vi "askForSerialNumber.vi"() -> (1 "Stop":bool, 2 "Setup":bool, 3 "Serial Number scanned":string)   [LabVIEW 2013]
panel:
  in  "Serial Number":string
  in  "OK Button":bool
  in  "Stop":bool
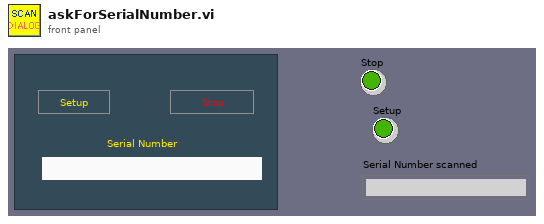
[diagram p1: front panel]
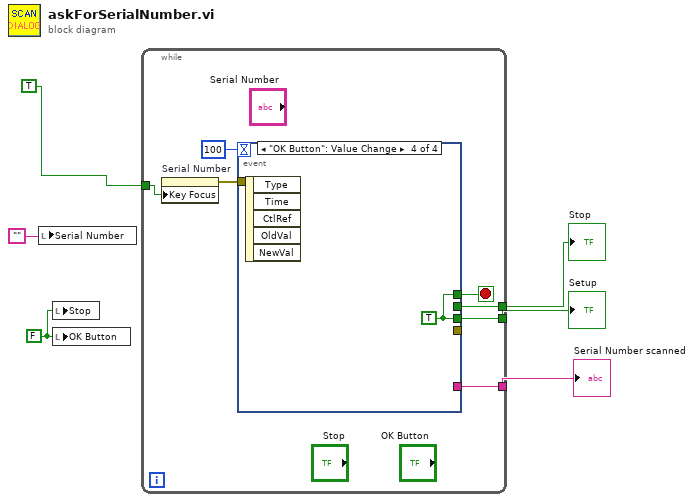
[diagram p0: block diagram]
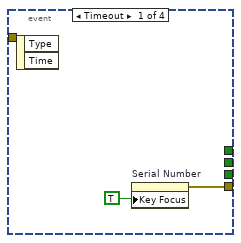
[diagram p2: hidden frame]
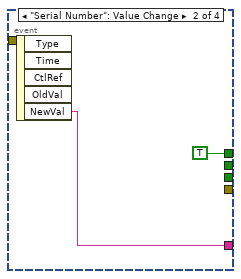
[diagram p3: hidden frame]
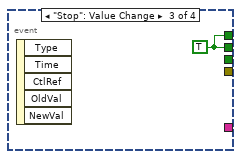
[diagram p4: hidden frame]
diagram:
  w4 = FALSE
  n1 = local write "Serial Number"("") -> ()
  n2 = local write "Stop"(w4) -> ()
  n3 = local write "OK Button"(w4) -> ()
  n4 = while {
    tunnel: [w12] -> w3
    tunnel: [w11] -> w6
    tunnel: [w10] -> w5
    tunnel: TRUE -> [w7]
    stop <- w9 stop-if-true
    n5 = property on="Serial Number" class="Str"("Key Focus"=w7) -> (error out=w8:errorcluster)  [unwired: 2 in, 1 out]
    n6 = event shown="[3] \"OK Button\": Value Change" {
      selector: _ -> [_ _ _ _]
      dyn-events: _ -> [_ _ _ _]
      timeout: 100 -> [_ _ _ _]
      tunnel: [_ _ w18 _] -> w12
      tunnel: [_ _ _ w19] -> w11
      tunnel: [_ w17 _ _] -> w10
      tunnel: [_ TRUE w18 w19] -> w9
      tunnel: [w15 _ _ _] -> _
      tunnel: w8 -> [_ _ _ _]
      event Timeout {
        n7 = event-data() -> ()  [unwired: 1 in, 2 out]
        n8 = property on="Serial Number" class="Str"("Key Focus"=TRUE) -> (error out=w15:errorcluster)  [unwired: 2 in, 1 out]
      }
      event "Serial Number": Value Change {
        n9 = event-data() -> ("NewVal"=w17:string)  [unwired: 1 in, 4 out]
      }
      event "Stop": Value Change {
        w18 = TRUE
        n10 = event-data() -> ()  [unwired: 1 in, 5 out]
      }
      event "OK Button": Value Change {
        w19 = TRUE
        n11 = event-data() -> ()  [unwired: 1 in, 5 out]
      }
    }
  }
  "Stop" <- w3
  "Setup" <- w6
  "Serial Number scanned" <- w5
